vi "Time Stamp to EPICS Time Stamp.vi"(0 "time stamp":timestamp, 1 "user tag":i32) -> (2 "EPICS time stamp":T1)   [LabVIEW 2020, in "PV Access.lvlib" / "PV Data.lvlib"]
uses:
  PV Data.lvlib
  EPICS Time Stamp.ctl
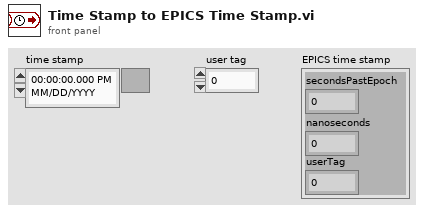
[diagram p1: front panel]
types:
  T1 = typedef "PV Access.lvlib/PV Data.lvlib/EPICS Time Stamp.ctl" = cluster{"secondsPastEpoch":i64, "nanoseconds":i32, "userTag":i32}
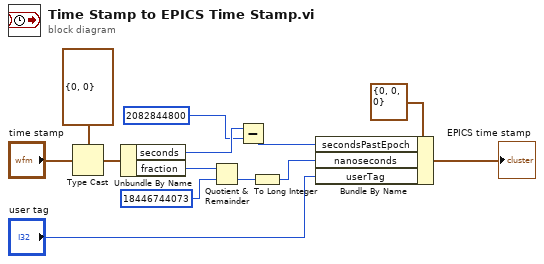
[diagram p0: block diagram]
diagram:
  n1 = Type Cast(type=cluster{"seconds":i64, "fraction":u64} {"seconds"=0, "fraction"=0}, x="time stamp") -> (*(type *) &x=w11:cluster{"seconds":i64, "fraction":u64})
  n2 = Unbundle By Name(w11) -> ("seconds"=w10:i64, "fraction"=w5:u64)
  n3 = Quotient & Remainder(x=w5, y=u64 18446744073) -> (floor(x/y)=w3:u64)  [unwired: 1 out]
  n4 = Subtract(x=w10, y=i64 2082844800) -> (x-y=w7:i64)
  n5 = To Long Integer(number=w3) -> (32bit integer=w2:i32)
  n6 = Bundle By Name(cluster=T1 {"secondsPastEpoch"=0, "nanoseconds"=0, "userTag"=0} ("timestamp"), "secondsPastEpoch"=w7, "nanoseconds"=w2, "userTag"="user tag") -> (→"EPICS time stamp":T1)
